vi "Serial Params--constant.vi"() -> (3 "Serial Configuration":T1={"Baud Rate"=9600, "Flow Control"=0, "Parity"=0, "Data Bits"=8} {"Baud Rate" items=["300"=300, "600"=600, "1200"=1200, "2400"=2400, "4800"=4800, "9600"=9600, "19200"=19200]; "Flow Control" items=["NONE", "SOFTWARE"]; "Parity" items=["NONE", "ODD", "EVEN"]; "Data Bits" items=["7"=7, "8"=8]})   [LabVIEW 2025]
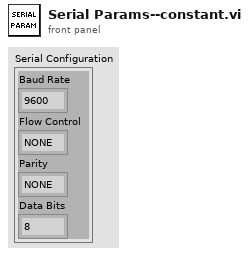
[diagram p1: front panel]
types:
  T1 = cluster{"Baud Rate":u32, "Flow Control":u16, "Parity":u16, "Data Bits":u16}
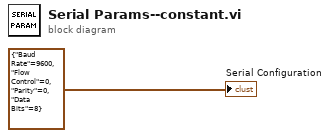
[diagram p0: block diagram]
diagram:
  "Serial Configuration" <- T1 {"Baud Rate"=9600, "Flow Control"=0, "Parity"=0, "Data Bits"=8} ("Serial Configuration")
